vi "Push.vi"(6 "Push Options":T1, 8 "error in (no error)":errorcluster, 9 "Refspecs":string[](array[string]), 10 "Repository":string, 11 "Git Implementation in":refnum<class "Git Implementation.lvclass">) -> (0 "error out":errorcluster, 2 "Status Message":string, 3 "Git Implementation out":refnum<class "Git Implementation.lvclass">)   [LabVIEW 2017, in "Git-LabVIEW.lvlib" / "Git Implementation.lvclass"]
doc: "Updates remote refs using local refs, while sending objects necessary to complete the given refs.\n\nRepository can be the name of a remote (e.g. \"origin\") or a URL. If it is empty, then the value is taken from the configuration for the local repository (via branch.*.remote). If no configuration exists, then \"origin\" is used)."
uses:
  Git Implementation.lvclass
  Push Options.ctl
  Force Mode.ctl
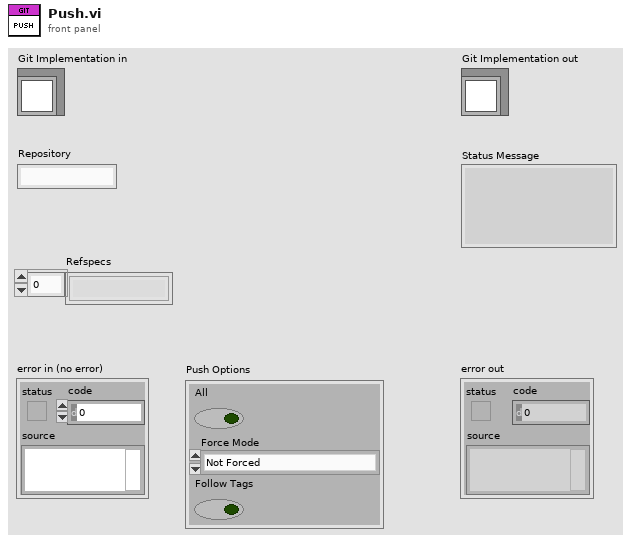
[diagram p1: front panel]
types:
  T1 = typedef "Git-LabVIEW.lvlib/Git Implementation.lvclass/Push Options.ctl" = cluster{"All":bool, "Force Mode":T2, "Follow Tags":bool}
  T2 = typedef "Git-LabVIEW.lvlib/Git Implementation.lvclass/Force Mode.ctl" = enum16{"Not Forced", "Force", "Force with Lease"}
  T3 = typedef "Git-LabVIEW.lvlib/Git Implementation.lvclass/CMD Return.ctl" = cluster{"StdOut":string, "StdErr":string, "Return Code":i32}
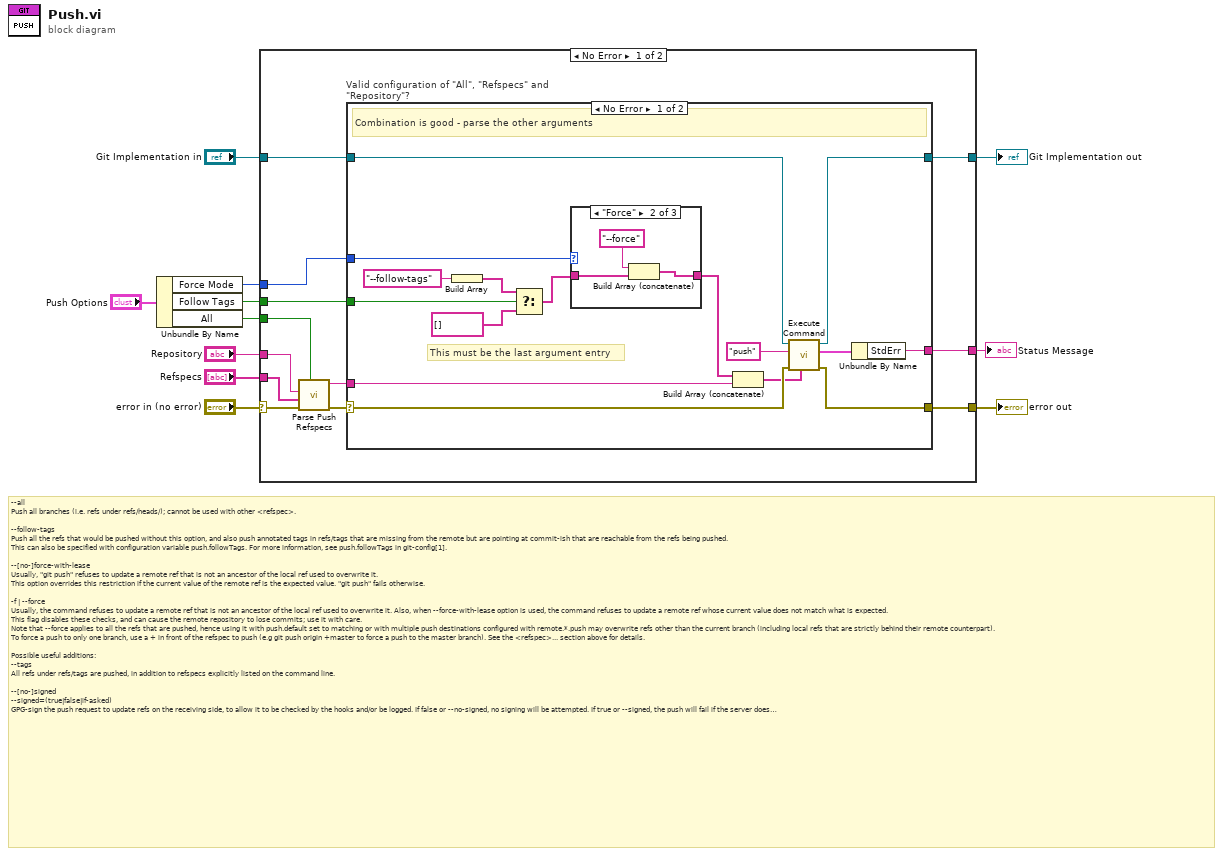
[diagram p0: block diagram]
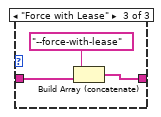
[diagram p3: hidden frame]
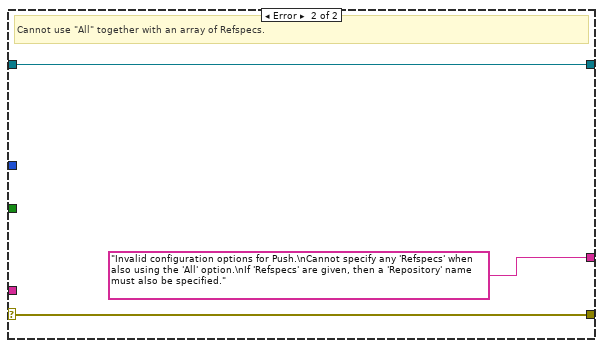
[diagram p4: hidden frame]
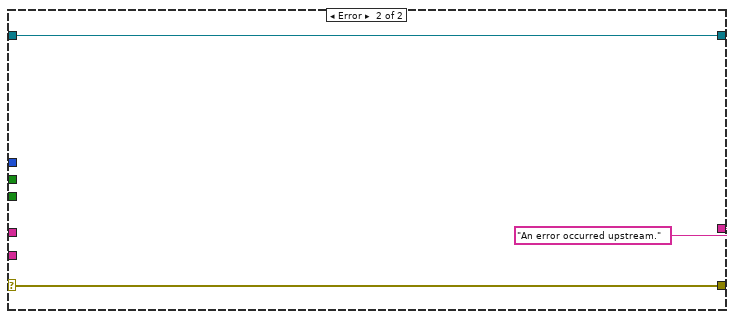
[diagram p5: hidden frame]
diagram:
  # "--all\nPush all branches (i.e. refs under refs/heads/); cannot be used with other <refspec>.\n\n--follow-tags\nPush all the refs that would be pushed without this option, and also push annotated tags in refs/tags that are missing from the remote but are pointing at commit-ish that are reachable from the refs being pushed. \nThis can also be specified with configuration variable push.followTags. For more information, see push.followTags in git-config[1].\n\n--[no-]force-with-lease\nUsually, \"git push\" refuses to update a remote ref that is not an ancestor of the local ref used to overwrite it.\nThis option overrides this restriction if the current value of the remote ref is the expected value. \"git push\" fails otherwise.\n\n-f | --force\nUsually, the command refuses to update a remote ref that is not an ancestor of the local ref used to overwrite it. Also, when --force-with-lease option is used, the command refuses to update a remote ref whose current value does not match what is expected.\nThis flag disables these checks, and can cause the remote repository to lose commits; use it with care.\nNote that --force applies to all the refs that are pushed, hence using it with push.default set to matching or with multiple push destinations configured with remote.*.push may overwrite refs other than the current branch (including local refs that are strictly behind their remote counterpart). \nTo force a push to only one branch, use a + in front of the refspec to push (e.g git push origin +master to force a push to the master branch). See the <refspec>... section above for details.\n\nPossible useful additions:\n--tags\nAll refs under refs/tags are pushed, in addition to refspecs explicitly listed on the command line.\n\n--[no-]signed\n--signed=(true|false|if-asked)\nGPG-sign the push request to update refs on the receiving side, to allow it to be checked by the hooks and/or be logged. If false or --no-signed, no signing will be attempted. If true or --signed, the push will fail if the server does not support signed pushes. \nIf set to if-asked, sign if and only if the server supports signed pushes. The push will also fail if the actual call to gpg --sign fails. See git-receive-pack[1] for the details on the receiving end.\n-u | --set-upstream\nFor every branch that is up to date or successfully pushed, add upstream (tracking) reference, used by argument-less git-pull[1] and other commands. For more information, see branch.<name>.merge in git-config[1].\n\n-q\n--quiet\nSuppress all output, including the listing of updated refs, unless an error occurs. Progress is not reported to the standard error stream.\n\n-v\n--verbose\nRun verbosely.\n\n--progress\nProgress status is reported on the standard error stream by default when it is attached to a terminal, unless -q is specified. This flag forces progress status even if the standard error stream is not directed to a terminal.\n\n--no-recurse-submodules\n--recurse-submodules=check|on-demand|only|no\nMay be used to make sure all submodule commits used by the revisions to be pushed are available on a remote-tracking branch. If check is used Git will verify that all submodule commits that changed in the revisions to be pushed are available on at least one remote of the submodule. \nIf any commits are missing the push will be aborted and exit with non-zero status. If on-demand is used all submodules that changed in the revisions to be pushed will be pushed. If on-demand was not able to push all necessary revisions it will also be aborted and exit with non-zero status. \nIf only is used all submodules will be recursively pushed while the superproject is left unpushed. A value of no or using --no-recurse-submodules can be used to override the push.recurseSubmodules configuration variable when no submodule recursion is required.\n\nThe options below are removed from this VI for simplicity - for further information about their functions read https://git-scm.com/docs/git-push\nIgnored Options:\n--mirror\n--dry-run | -n\n--porcelain\n--delete\n--[no-]atomic\n--push-option=<option> | -o <option>\n--receive-pack=<git-receive-pack>\n--exec=<git-receive-pack>\n--force-with-lease=<...> (the version without additional arguments is implemented via the \"Force Mode\" enum)\n--repo=<repository> (implemented via \"Repository\" string control)\n--[no-]thin\n--ipv4 | -4, --ipv6 | -6"
  n1 = Unbundle By Name("Push Options") -> ("Force Mode"=w3:T2, "Follow Tags"=w2:bool, "All"=w1:bool)
  n2 = case shown="No Error" "error in (no error)" {
    selector: "error in (no error)" -> [w17 w52]
    tunnel: [w23 w52] -> w10
    tunnel: [w21 w51] -> w8
    tunnel: "Git Implementation in" -> [w22 w51]
    tunnel: "Refspecs" -> [w18 _]
    tunnel: "Repository" -> [w19 _]
    tunnel: [w20 "An error occurred upstream." ("StdOut")] -> w5
    tunnel: w1 -> [w12 _]
    tunnel: w3 -> [w14 _]
    tunnel: w2 -> [w13 _]
    frame No Error {
      n3 = call "Parse Push Refspecs.vi"("All"=w12, "error in (no error)"=w17, "Refspecs"=w18, "Repository"=w19) -> ("error out"=w16:errorcluster, "Final Argument String"=w15:string)  [unwired: 6 in]
      n4 = case "Valid configuration of \"All\", \"Refspecs\" and \"Repository\"?" shown="No Error" w16 {
        selector: w16 -> [w32 w47]
        tunnel: [w39 w47] -> w23
        tunnel: w22 -> [w37 w49]
        tunnel: [w36 w49] -> w21
        tunnel: [w34 "Invalid configuration options for Push.\nCannot specify any 'Refspecs' when also using the 'All' option.\nIf 'Refspecs' are given, then a 'Repository' name must also be specified." ("StdErr")] -> w20
        tunnel: w15 -> [w33 _]
        tunnel: w14 -> [w31 _]
        tunnel: w13 -> [w28 _]
        frame No Error {
          # "This must be the last argument entry"
          # "Combination is good - parse the other arguments"
          n5 = Build Array("--follow-tags" ("Final Argument String")) -> (w25:string[])
          n6 = Select(t=w25, s=w28, f=string[] []) -> (s? t:f=w24:string[])
          n7 = case shown="\"Force\"" w31 {
            tunnel: w24 -> [w40 w43 w46]
            tunnel: [w40 w41 w44] -> w29
            frame "Not Forced" {
            }
            frame "Force" {
              n8 = Build Array (concatenate)("--force", w43) -> (w41:string[])
            }
            frame "Force with Lease" {
              n9 = Build Array (concatenate)("--force-with-lease", w46) -> (w44:string[])
            }
          }
          n10 = Build Array (concatenate)(w29, w33) -> (w30:string[])
          n11 = call "Execute Command.vi"("Arguments"=w30, "error in (no error)"=w32, "Command"="push", "Git Implementation in"=w37) -> ("error out"=w39:errorcluster, "CMD Return"=w35:T3, "Git Implementation out"=w36:refnum<class "Git Implementation.lvclass">)  [unwired: 5 in]
          n12 = Unbundle By Name(w35) -> ("StdErr"=w34:string)
        }
        frame Error {
          # "Cannot use \"All\" together with an array of Refspecs."
        }
      }
    }
    frame Error {
    }
  }
  "error out" <- w10
  "Git Implementation out" <- w8
  "Status Message" <- w5
